vi "grab.vi"(8 "error in (no error)":errorcluster, 9 "buf in":u16[][](array[numeric]), 10 "Mbuf":refnum<k24>, 11 ".NET Refnum in":refnum<k24>) -> (0 "error out":errorcluster, 2 "Image Out":T1, 3 ".NET Refnum out":refnum<k24>)   [LabVIEW 2019]
uses:
  <vilib>/vision/Image Controls.llb/IMAQ Image.ctl
  C:/Users/huang/Desktop/MIL LITE 10/64/Matrox Imaging/MIL/MIL.NET/Matrox.MatroxImagingLibrary.v3.5.dll
  64/Matrox Imaging/MIL/MIL.NET/Matrox.MatroxImagingLibrary.v3.5.dll
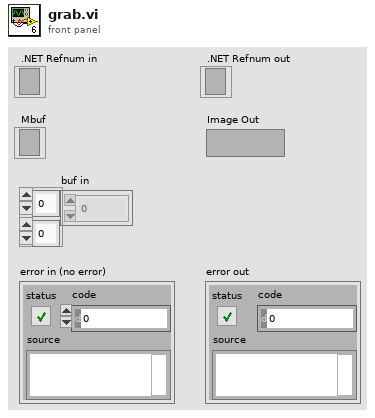
[diagram p1: front panel]
types:
  T1 = typedef "IMAQ Image.ctl" = refnum<image>
  T2 = typedef "Image Type" = u32
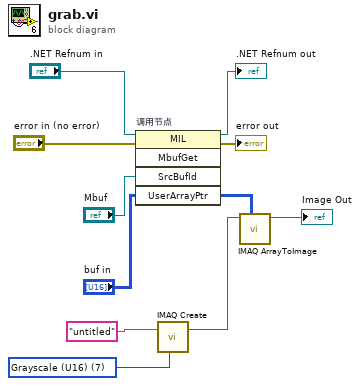
[diagram p0: block diagram]
diagram:
  w8 = T2 7 items=["Grayscale (U8)", "Grayscale (I16)", "Grayscale (SGL)", "Complex (CSG)", "RGB (U32)", "HSL (U32)", "RGB (U64)", "Grayscale (U16)"] ("Image Type")
  n1 = invoke on="调用节点" class="MIL" method="MbufGet"(reference=".NET Refnum in", error in="error in (no error)", "SrcBufId"="Mbuf", "UserArrayPtr"="buf in") -> (reference out=→".NET Refnum out":refnum<k24>, error out=→"error out":errorcluster, "UserArrayPtr"=w10:u16[][])  [unwired: 1 in, 2 out]
  n2 = call "IMAQ Create"("Image Name"="untitled", "Image Type"=w8) -> ("New Image"=w9:T1)  [unwired: 3 in, 1 out]
  n3 = call "IMAQ ArrayToImage"("Image Pixels (U16)"=w10, "Image"=w9) -> ("Image Out"=→"Image Out":T1)  [unwired: 8 in, 1 out]
